vi "Find Owning VI Target Item.vi"(11 "viref":refnum<vi>) -> (3 "targetItem":refnum<vi>)   [LabVIEW 2020, in "NI_TargetHelper.lvlib"]
uses:
  <vilib>/TargetSupport/NI_TargetHelper/NI_TargetHelper.lvlib
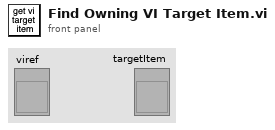
[diagram p1: front panel]
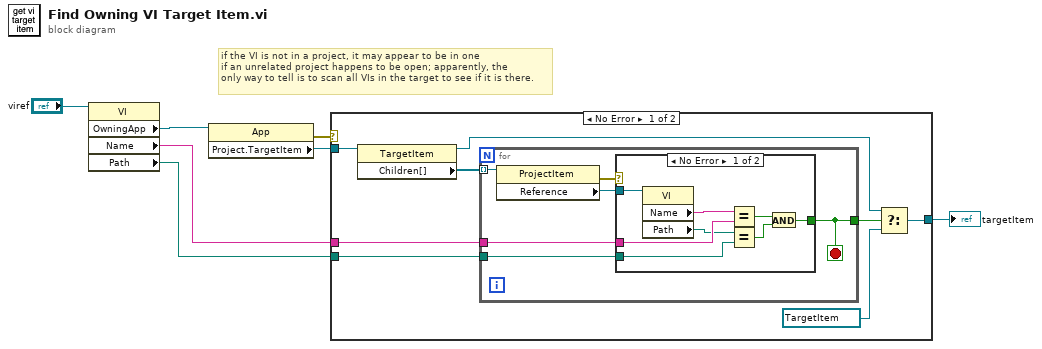
[diagram p0: block diagram]
diagram:
  # "if the VI is not in a project, it may appear to be in one\nif an unrelated project happens to be open; apparently, the \nonly way to tell is to scan all VIs in the target to see if it is there."
  n1 = property class="VI"(reference="viref") -> ("OwningApp"=w7:refnum<vi>, "Name"=w3:string, "Path"=w2:path)  [unwired: 1 in, 2 out]
  n2 = property class="App"(reference=w7) -> (error out=w4:errorcluster, "Project.TargetItem"=w6:refnum<vi>)  [unwired: 1 in, 1 out]
  n3 = case shown="No Error" w4 {
    tunnel: w6 -> [w15 _]
    tunnel: w3 -> [w13 _]
    tunnel: w2 -> [w12 _]
    tunnel: [w8 _] -> w1
    frame No Error {
      n4 = property class="TargetItem"(reference=w15) -> (reference out=w10:refnum<vi>, "Children[]"=w14:refnum<vi>[])  [unwired: 1 in, 1 out]
      n5 = for {
        tunnel: w14 -> [w21] mode=indexing
        tunnel: w13 -> [w19]
        tunnel: w12 -> [w18]
        tunnel: [w16] -> w11
        stop <- w16 stop-if-true
        n6 = property class="ProjectItem"(reference=w21) -> (error out=w17:errorcluster, "Reference"=w20:refnum<vi>)  [unwired: 1 in, 1 out]
        n7 = case shown="No Error" w17 {
          tunnel: w20 -> [w29 _]
          tunnel: w19 -> [w27 _]
          tunnel: w18 -> [w25 _]
          tunnel: [w22 _] -> w16
          frame No Error {
            n8 = property class="VI"(reference=w29) -> ("Name"=w28:string, "Path"=w26:path)  [unwired: 1 in, 2 out]
            n9 = Equal?(x=w28, y=w27) -> (x = y?=w23:bool)
            n10 = Equal?(x=w26, y=w25) -> (x = y?=w24:bool)
            n11 = And(x=w23, y=w24) -> (x .and. y?=w22:bool)
          }
          frame Error {
          }
        }
      }
      n12 = Select(t=w10, s=w11, f=refnum<vi> refnum ("t")) -> (s? t:f=w8:refnum<vi>)
    }
    frame Error {
    }
  }
  "targetItem" <- w1
